vi "Start Temperature.vi"(0 "reference in":refnum<class "Temp.lvclass">, 5 "error in (no error)":errorcluster) -> (14 "reference out":refnum<class "Temp.lvclass">, 19 "error out":errorcluster)   [LabVIEW 2017, in "Temp.lvclass"]
uses:
  Temp.lvclass
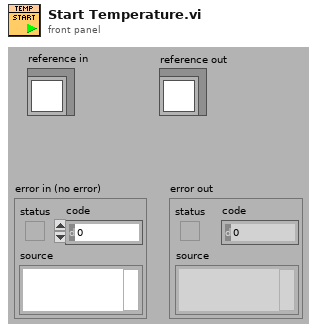
[diagram p1: front panel]
types:
  T1 = typedef "Temp.lvclass/ObjectAttributes.ctl" = cluster{"Temperature Task":refnum<k21>, "Temperature Readings":dbl[], "Thermocouple Type":i32, "Temperature Units":i32, "Average Temperature":dbl, "Number of Temperature Modules":i32, "Number of Total Temperature Channels":i32, "Temperature On/Off Status":bool, "Temperature Module Names (NI-Max Name)":string[], "Number of Channels Per Temperature  Module":i32[], "Temperature VI Reference":refnum<vi>}
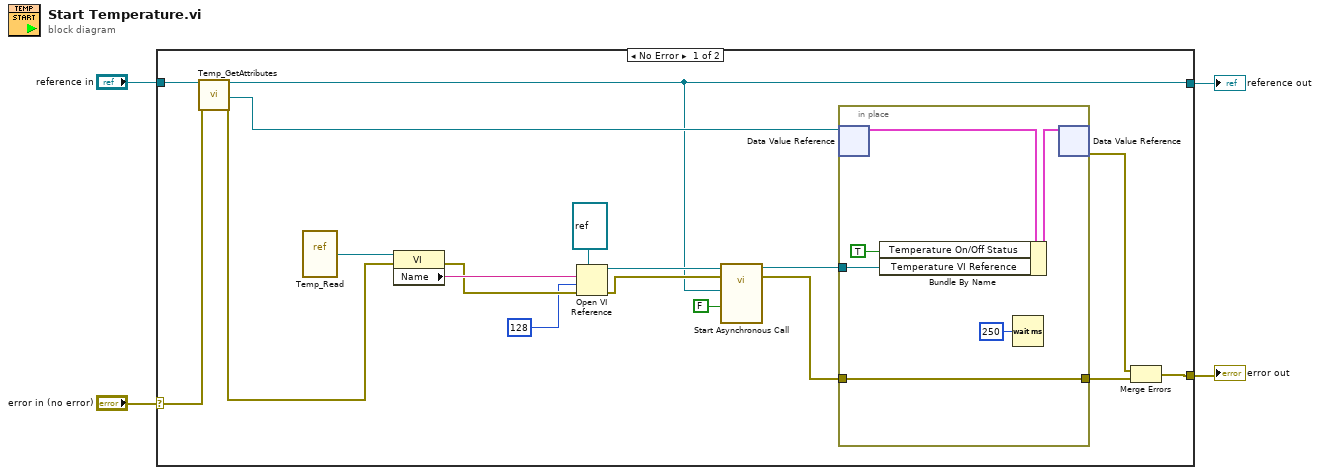
[diagram p0: block diagram]
diagram:
  n1 = case shown="No Error" "error in (no error)" {
    selector: "error in (no error)" -> [w21 w30]
    tunnel: [w19 w30] -> w3
    tunnel: [w8 w29] -> w1
    tunnel: "reference in" -> [w22 w29]
    frame No Error {
      n2 = call "Temp_GetAttributes.vi"("reference in"=w22, "error in (no error)"=w21) -> ("reference out"=w8:refnum<class "Temp.lvclass">, "DataRef"=w18:refnum<data-value>, "error out"=w5:errorcluster)  [unwired: 14 in, 1 out]
      n3 = vi-ref "Temp_Read.vi"() -> (w15:refnum<vi>)
      n4 = property class="VI"(reference=w15, error in=w5) -> (error out=w14:errorcluster, "Name"=w16:string)  [unwired: 1 out]
      n5 = Open VI Reference(type specifier VI Refnum (for type only)=refnum<vi> refnum, vi path=w16, options=128, error in (no error)=w14) -> (vi reference=w11:refnum<vi>, error out=w10:errorcluster)  [unwired: 2 in]
      n6 = call-by-ref "Start Asynchronous Call"(reference=w11, error in=w10, "Stop Temperature"=FALSE, "reference in"=w8) -> (reference out=w7:refnum<vi>, error out=w6:errorcluster)  [unwired: 8 in, 2 out]
      n7 = in-place {
        in-place-border: w6 -> [w26]
        in-place-border: [w26] -> w17
        in-place-border: w7 -> [w24]
        n8 = in-place-dvr #1(w18) -> (w27:T1)  [unwired: 1 out]
        n9 = Bundle By Name(cluster=w27, "Temperature On/Off Status"=TRUE, "Temperature VI Reference"=w24) -> (w28:T1)
        n10 = Wait (ms)(milliseconds to wait=u32 250) -> ()  [unwired: 1 out]
        n11 = in-place-dvr #1(w28) -> (w20:errorcluster)  [unwired: 1 out]
      }
      n12 = Merge Errors(w20, w17) -> (w19:errorcluster)
    }
    frame Error {
    }
  }
  "error out" <- w3
  "reference out" <- w1
